vi "Process.vi"(8 "error in (no error)":errorcluster, 10 "Wash Abort Terminate State in":refnum<class "Wash Abort Terminate State.lvclass">, 11 "Architecture.lvlib:Thread.lvclass":refnum<class "Thread.lvclass">) -> (0 "error out":errorcluster, 1 "Stop?":bool, 3 "Architecture.lvlib:Thread.lvclass 2":refnum<class "Thread.lvclass">)   [LabVIEW 2012, in "Car Wash Controller.lvlib" / "Wash Abort Terminate State.lvclass"]
uses:
  Wash Abort Terminate State.lvclass
  Message/Message.lvclass
  Thread/Thread.lvclass
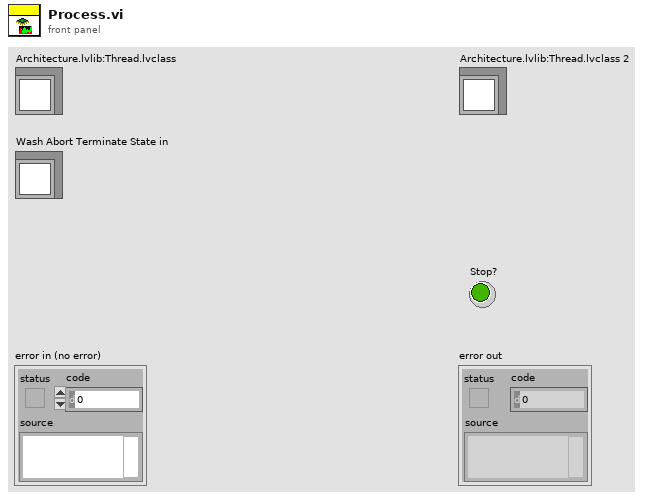
[diagram p1: front panel]
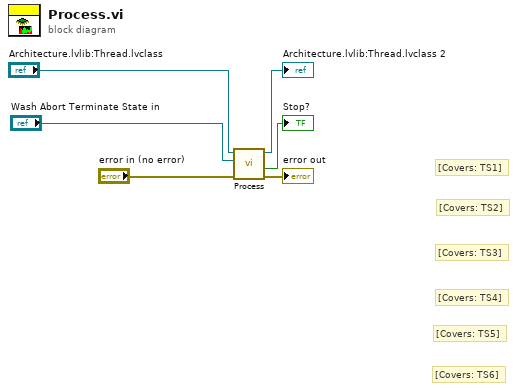
[diagram p0: block diagram]
diagram:
  # "[Covers: TS6]"
  # "[Covers: TS5]"
  # "[Covers: TS4]"
  # "[Covers: TS3]"
  # "[Covers: TS2]"
  # "[Covers: TS1]"
  n1 = call-parent "Process.vi"("error in (no error)"="error in (no error)", "Message in"="Wash Abort Terminate State in", "Architecture.lvlib:Thread.lvclass"="Architecture.lvlib:Thread.lvclass") -> ("error out"=→"error out":errorcluster, "Stop?"=→"Stop?":bool, "Architecture.lvlib:Thread.lvclass 2"=→"Architecture.lvlib:Thread.lvclass 2":refnum<class "Thread.lvclass">)  [unwired: 6 in]
